vi "PH_BL-Master.Find Picture GUI Ref by Name.vi"(2 "Pic Ref Array":refnum<vi>[](array[refnum]), 4 "Label":string, 5 "error in":errorcluster) -> (16 "Wanted Pic GUI Ref":refnum<vi>, 17 "Ref found?":bool, 18 "index of element":i32, 19 "error out":errorcluster)   [LabVIEW 2014, in "PH_BL-Master.lvlib"]
uses:
  PH_BL-Master.lvlib
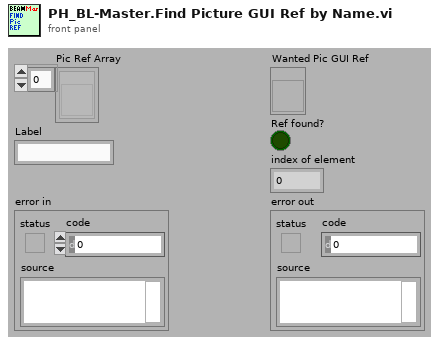
[diagram p1: front panel]
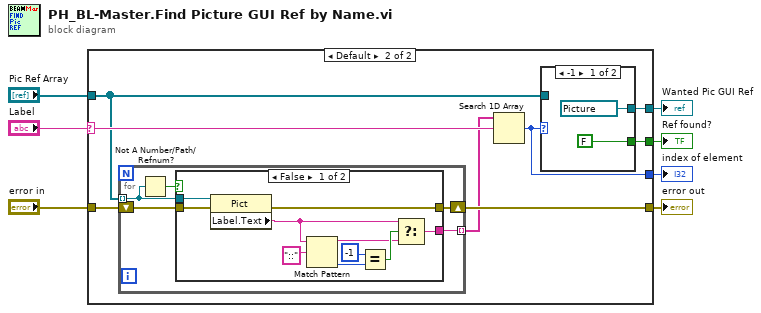
[diagram p0: block diagram]
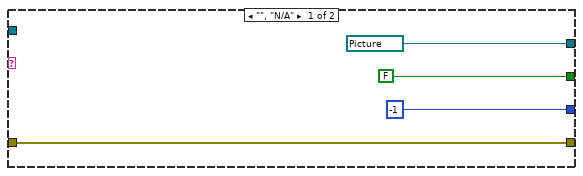
[diagram p2: hidden frame]
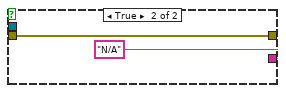
[diagram p3: hidden frame]
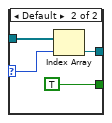
[diagram p4: hidden frame]
diagram:
  n1 = case shown="Default" "Label" {
    selector: "Label" -> [_ w16]
    tunnel: [refnum<vi> refnum ("Pic GUI Ref") w19] -> w7
    tunnel: [-1 ("index of element") w18] -> w6
    tunnel: [FALSE w17] -> w5
    tunnel: "Pic Ref Array" -> [_ w12]
    tunnel: "error in" -> [w11 w15]
    tunnel: [w11 w14] -> w2
    frame "", "N/A" {
    }
    frame Default {
      n2 = for {
        tunnel: w12 -> [w20] mode=indexing
        tunnel: [w24] -> w13 mode=indexing
        shift-right: [w23] -> w14
        shift-left: w15 -> [w22]
        n3 = Not A Number/Path/Refnum?(number/path/refnum=w20) -> (NaN/Path/Refnum?=w21:bool)
        n4 = case shown="False" w21 {
          tunnel: w20 -> [w34 _]
          tunnel: [w28 "N/A" ("Label.Text")] -> w24
          tunnel: [w33 w35] -> w23
          tunnel: w22 -> [w32 w35]
          frame False {
            n5 = property class="Pict"(reference=w34, error in=w32) -> (error out=w33:errorcluster, "Label.Text"=w29:string)  [unwired: 1 out]
            n6 = Match Pattern(string=w29, regular expression="::") -> (before substring=w27:string, offset past match=w26:i32)  [unwired: 1 in, 2 out]
            n7 = Equal?(x=-1 ("y"), y=w26) -> (x = y?=w30:bool)
            n8 = Select(t=w29, s=w30, f=w27) -> (s? t:f=w28:string)
          }
          frame True {
          }
        }
      }
      n9 = Search 1D Array(1D array=w13, element=w16) -> (index of element=w18:i32)  [unwired: 1 in]
      n10 = case shown="-1" w18 {
        selector: w18 -> [_ w40]
        tunnel: w12 -> [_ w42]
        tunnel: [refnum<vi> refnum ("CH Ref") w41] -> w19
        tunnel: [FALSE TRUE] -> w17
        frame -1 {
        }
        frame Default {
          n11 = Index Array(array=w42, index=w40) -> (element=w41:refnum<vi>)
        }
      }
    }
  }
  "error out" <- w2
  "Wanted Pic GUI Ref" <- w7
  "Ref found?" <- w5
  "index of element" <- w6
